vi "REFERECNE Dashboard Main.vi"() -> ()   [LabVIEW 2023]
uses:
  Shared Code/TypeDefs/ENUM RB_Drive Mode IND.ctl
  Shared Code/TypeDefs/Cluster_CMD_Direction Data.ctl
  Shared Code/TypeDefs/Cluster_Module Velocity-Direction-Rotations.ctl
  Shared Code/TypeDefs/Level_Velocity plus-minus 1.ctl
  Shared Code/TypeDefs/Dial_Compase heading unit circle CCW positive.ctl
  Shared Code/TypeDefs/ENUM RB_Feeder State.ctl
  Support/Utility/FP_Size VI to Decoration Simple.vi/TypeDefs_Utility/Cluster_FP Set.ctl
  Support/Utility/FP_Size VI to Decoration Simple.vi/TypeDefs_Utility/ENUM RB_Pos_Quadrant Position.ctl
  <vilib>/event_ctls.llb/eventvkey.ctl
  <vilib>/Utility/miscctls.llb/LVForegroundBackgroundColorsTypeDef.ctl
  dc37a527-230c-42ca-8007-a2fc15904402.vi
  b20e14a2-edb0-4227-a406-03726573f279.vi
  <vilib>/Rock Robotics/Network Tables/NT Read Numeric Array.vi
  <vilib>/Rock Robotics/WPI/Dashboard/WPI_DashboardLogging Global.vi
panel:
  in  "Camera Settings Right":T1={"Frame Rate"=30, "Compression"=30, "Size"=1, "DB Camera Config"=FALSE} {"Frame Rate" scale=1.0..30.0; "Compression" scale=100.0..-1.0; "Size" items=["640x480", "320x240", "160x120"]}
  in  "Camera Name Right":string(combo)="No Camera Selection"
  out "Camera Perf":string
  in  "Camera Settings":T1={"Frame Rate"=30, "Compression"=30, "Size"=1, "DB Camera Config"=FALSE} {"Frame Rate" scale=1.0..30.0; "Compression" scale=100.0..-1.0; "Size" items=["640x480", "320x240", "160x120"]}
  in  "TCP":refnum<k5>
  out "Robot IP":string
  out "Image Message":string="Timeout in Camera Communications"
  in  "Dashboard Tab":T2(tab)=enum."Custom"
  in  "Select Auto":string(combo)="Select Autonomous ..."
  out "NT Connection":bool
  out "MotorChart R":cluster{"Numeric":dbl, "Numeric":dbl}(graph)
  out "MotorChart L":cluster{"Numeric":dbl, "Numeric":dbl}(graph)
  out "MotorSliders R":cluster{"MotorSlide1":dbl, "MotorSlide2":dbl} {"MotorSlide2" scale=-1.0..1.0 scale format="%#_2e"; "MotorSlide1" scale=-1.0..1.0 scale format="%#_2e"}
  out "MotorSliders L":cluster{"MotorSlide1":dbl, "MotorSlide2":dbl} {"MotorSlide2" scale=-1.0..1.0 scale format="%#_2e"; "MotorSlide1" scale=-1.0..1.0 scale format="%#_2e"}
  out "JS1 Z":dbl(slide) scale=-1.0..1.0 scale format="%#_2e"
  out "JS1 Graph":cluster{"X":dbl, "Y":dbl}[](graph)
  out "JS1 Buttons":T3
  out "JS2 Z":dbl(slide) scale=-1.0..1.0 scale format="%#_2e"
  out "JS2 Graph":cluster{"X":dbl, "Y":dbl}[](graph)
  out "JS2 Buttons":T3
  out "Mode":T4(ring)=enum."Auto Disabled"
  out "Right Camera Perf":cluster{"Bandwidth (Mbps)":dbl, "FPS":dbl}
  out "Camera Image Right":T5(plugin-control)
  in  "DB/String 9":string
  in  "DB/String 8":string
  in  "DB/String 7":string
  in  "DB/String 6":string
  in  "DB/String 5":string
  in  "DB/String 4":string
  in  "DB/String 3":string
  in  "DB/String 2":string
  in  "DB/String 1":string
  in  "DB/String 0":string
  in  "DB/Slider 0":dbl(slide) scale=0.0..5.0
  in  "DB/Slider 1":dbl(slide) scale=0.0..5.0
  in  "DB/Slider 2":dbl(slide) scale=0.0..5.0
  in  "DB/Slider 3":dbl(slide) scale=0.0..5.0
  out "DB/LED 3":bool
  out "DB/LED 2":bool
  out "DB/LED 1":bool
  out "DB/LED 0":bool
  in  "DB/Button 3":bool
  in  "DB/Button 2":bool
  in  "DB/Button 1":bool
  in  "DB/Button 0":bool caption="New Name"
  in  "Max Speed (FPS)":dbl(slide)=2.0 min=0.0 max=10.0 step=0.1 scale=0.0..10.0
  out "Tube":string
  out "Drive State":bool=TRUE
  out "Feeder State":T6
  out "Shooter Speed":cluster{dbl, dbl, dbl}(slide) scale=0.0..4500.0 scale format="%#.0f"
  out "Compass":T7 scale format="%.3f"
  out "Comand Data":T8 {"Rotate(Yaw) CCW 1 CW -1" scale=1.0..-1.0; "Traverse"."Angle" scale format="%.3f"; "Traverse"."Velocity" scale=-1.0..1.0 scale format="%.1f"}
  out "Robot MODE":T11
  in  "CheckList":i32(listbox)
  out "Tree":string(tree)
  out "Camera Image":T5(plugin-control)
  out "Background":bool
  in  "Camera Name":string(combo)="No Camera Selection"
  # "HW"
  # "HW"
  # "Joysticks"
  # "Drive Motors"
  # "Front"
  # "Right"
  # "Left"
  # "Back"
  # "Setting"
  # "Right"
  # "Left"
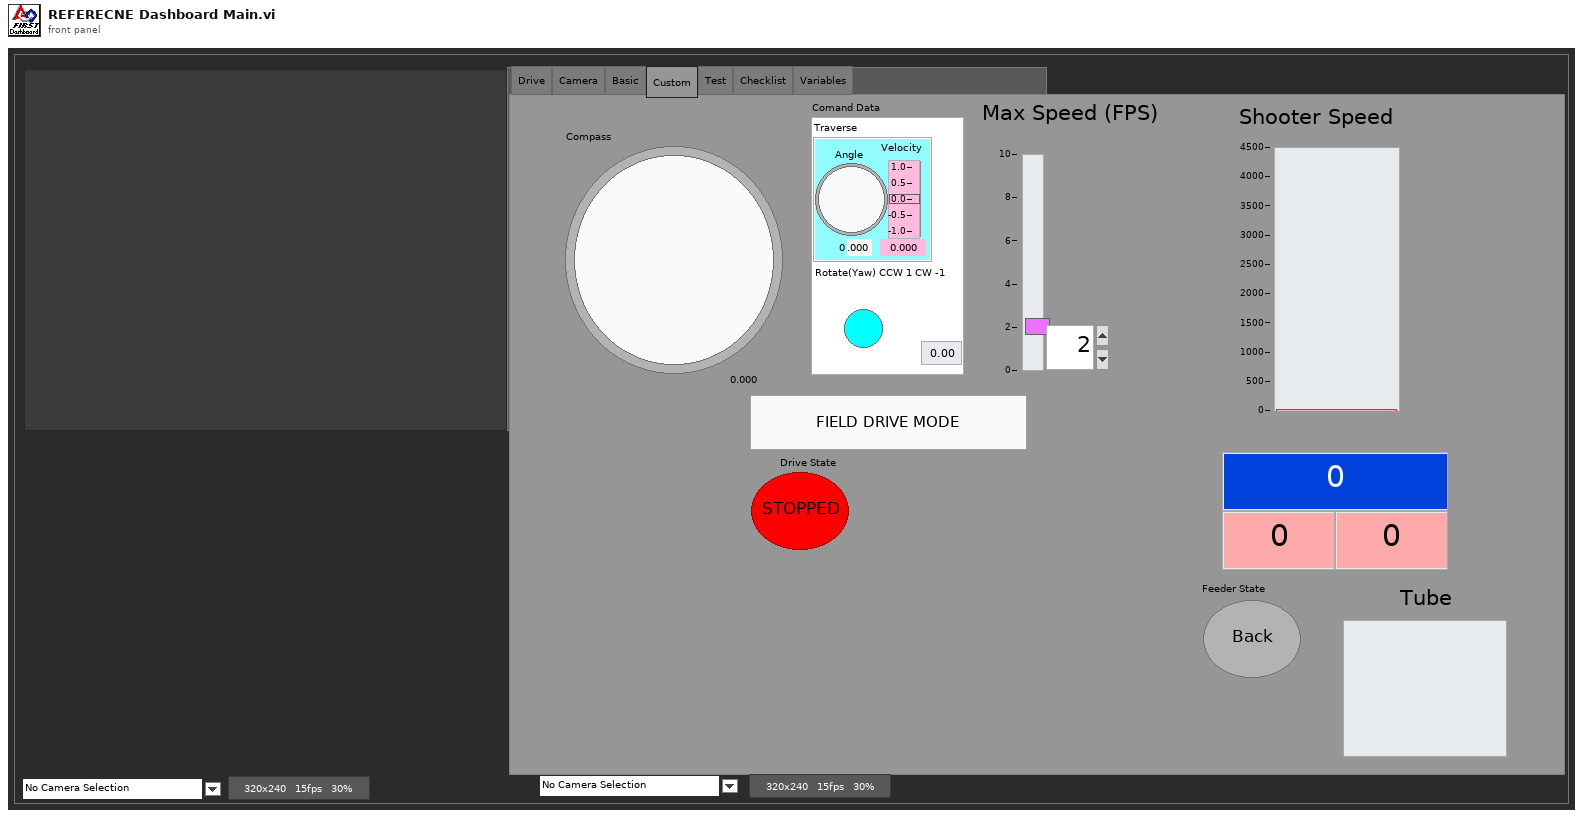
[diagram p1: front panel]
types:
  T1 = cluster{"Frame Rate":i32, "Compression":i32, "Size":u16, "DB Camera Config":bool}
  T2 = enum32{"Drive", "Camera", "Basic", "Custom", "Test", "Checklist", "Variables"}
  T3 = cluster{bool, bool, bool, bool, bool, bool, bool, bool, bool, bool, bool, bool}
  T4 = enum8{"Tele-Op Disabled", "Tele-Op Enabled", "Auto Disabled", "Auto Enabled", "Test Disabled", "Test Enabled", "Disconnected", "No Code", "E-Stop"}
  T5 = typedef "IMAQ Image.ctl" = refnum<image>
  T6 = typedef "ENUM RB_Feeder State.ctl" = enum32{"Back", "Reversing", "Shooting"}
  T7 = typedef "Dial_Compase heading unit circle CCW positive.ctl" = dbl
  T8 = typedef "Cluster_CMD_Direction Data.ctl" = cluster{"Traverse":T9, "Rotate(Yaw) CCW 1 CW -1":dbl}
  T9 = typedef "Cluster_Module Velocity-Direction-Rotations.ctl" = cluster{"Velocity":T10, "Angle":T7, "Rotations Count":dbl}
  T10 = typedef "Level_Velocity plus-minus 1.ctl" = dbl
  T11 = typedef "ENUM RB_Drive Mode IND.ctl" = enum32{"Field Drive Mode", "Robot Drive Mode", "Turrent Drive Mode"}
  T12 = typedef "Cluster_FP Set.ctl" = cluster{"Menu Bar":bool, "Position":T13, "Decoration index":i32, "border(px)":i32, "Monitor #":i32}
  T13 = typedef "ENUM RB_Pos_Quadrant Position.ctl" = enum32{"LFT-TOP", "MID-TOP", "RGT-TOP", "LFT-CTR", "MID-CTR", "RGT-CTR", "LFT-BOT", "MID-BOT", "RGT-BOT"}
  T14 = cluster{"Save Path":path, "Interval (s)":dbl, "Keep":i32}
  T15 = enum32{"Drive", "Camera", "Basic", "Custom", "Test", "Commands", "Checklist", "Variables"}
  T16 = typedef "Image Type" = u32
  T17 = typedef "LVForegroundBackgroundColorsTypeDef.ctl" = cluster{"Foreground Color":u32, "Background Color":u32}
  T18 = cluster{"Error Strings":string, "Disable Counts":cluster{u16, u16}, "Rail Faults":cluster{u16, u16, u16}, "Robot IP":string, "DB Mode":u8, "Event Info":cluster{"Name":string, "Type":u8, "Number":u16, "Replay":u8}}
  T19 = cluster{"Storage":cluster{"Disk Free":u64, "RAM Block":u32, "RAM free":u32}, "CPU Utilization":cluster{"CPU % ISR":sgl, "CPU % Time Crit":sgl, "CPU % Timed Str":sgl, "CPU % High":sgl, "CPU % Above":sgl, "CPU % Normal":sgl, "CPU % Low":sgl}, "CAN":cluster{"% Bus Utilization":sgl, "Bus Off Cnt":u32, "TX_FIFO Full Cnt":u32, "Receive Error Cnt":u8, "Transmit Error Cnt":u8}, "HID":cluster{"HID Outputs":u32, "Rumble Low":u16, "Rumble High":u16}[]}
  T20 = cluster{"Status bits":cluster{"Test Mode":bool, "Autonomous":bool, "Enabled":bool, "Code Start":bool, "Brownout":bool, "Reserved 2":bool, "Reserved 3":bool, "E-Stop":bool}, "Code Trace":cluster{"Disabled":bool, "TeleOp":bool, "Auto":bool, "Test":bool}, "Controller Type":enum16{"unknown", "cRIO", "roboRio"}, "Code?":enum16{"unknown", "noCode", "code"}, "Battery V":dbl}
  T21 = cluster{"Control Bits":cluster{"TestMode":bool, "Autonomous":bool, "Enabled":bool, "FMS Present":bool, bool, bool, bool, "E-Stop":bool}, "Team Station ":u8, "Countdown":sgl, "Joystick Values":cluster{"Axes":dbl[], "Buttons":bool[], "POVs":i16[]}[]}
  T22 = typedef "Cluster_Shooter Speed Data.ctl" = cluster{"Set":dbl, "Left":dbl, "Right":dbl}
  T23 = typedef "ENUM_Tube Wheel Positions.ctl" = enum16{"Unknown-None", "Tube Red A", "Tube Black B", "Tube Red C", "Tube Black D", "Tube Red E", "Tube Black F", "Load A-B", "Load B-C", "Load C-D", "Load D-E", "Load E-F", "Load F-A"}
  T24 = cluster{"Axes":dbl[], "Buttons":bool[], "POVs":i16[]}[]
  T25 = cluster{"Axes":dbl[], "Buttons":bool[], "POVs":i16[]}
  T26 = cluster{"Buttons[0]":bool, "Buttons[1]":bool, "Buttons[2]":bool, "Buttons[3]":bool, "Buttons[4]":bool, "Buttons[5]":bool, "Buttons[6]":bool, "Buttons[7]":bool, "Buttons[8]":bool, "Buttons[9]":bool, "Buttons[10]":bool, "Buttons[11]":bool}
  T27 = cluster{"Global Rectangle":i32[], "Contours":cluster{"Contour Type":u32, "ROI Type":u32, "Points":i32[]}[]}
  T28 = cluster{"Camera Name Right":string, string, "Saved DB Images Info":cluster{"Save Path":path, "Interval (s)":dbl, "Keep":i32}}
  T29 = cluster{"Camera Name":string, string, "Saved DB Images Info":cluster{"Save Path":path, "Interval (s)":dbl, "Keep":i32}}
  T30 = cluster{"Operation":enum16{"Update", "Clear"}, "Color Box":u32}[]
  T31 = typedef "eventvkey.ctl" = enum16{"ASCII", "Enter", "Return", "Shift", "Ctrl", "Alt", "Cmd", "Opt", "Caps", "NumLock", "Clear", "Break", "Up", "Down", "Left", "Right", "Insert", "Delete", "Home", "End", "PageUp", "PageDown", "Escape", "Help", "Pause", "ScrollLock", "F1", "F2", "F3", "F4", "F5", "F6", "F7", "F8", "F9", "F10", "F11", "F12", "F13", "F14", "F15", "F16", "F17", "F18", "F19", "F20", "F21", "F22", "F23", "F24", "Play", "VolumeUp", "VolumeDown", "Mute", "Two Byte Char"}
  T32 = cluster{"Shift":bool, "Ctrl":bool, "Alt":bool, "Cmd":bool, "Opt":bool}
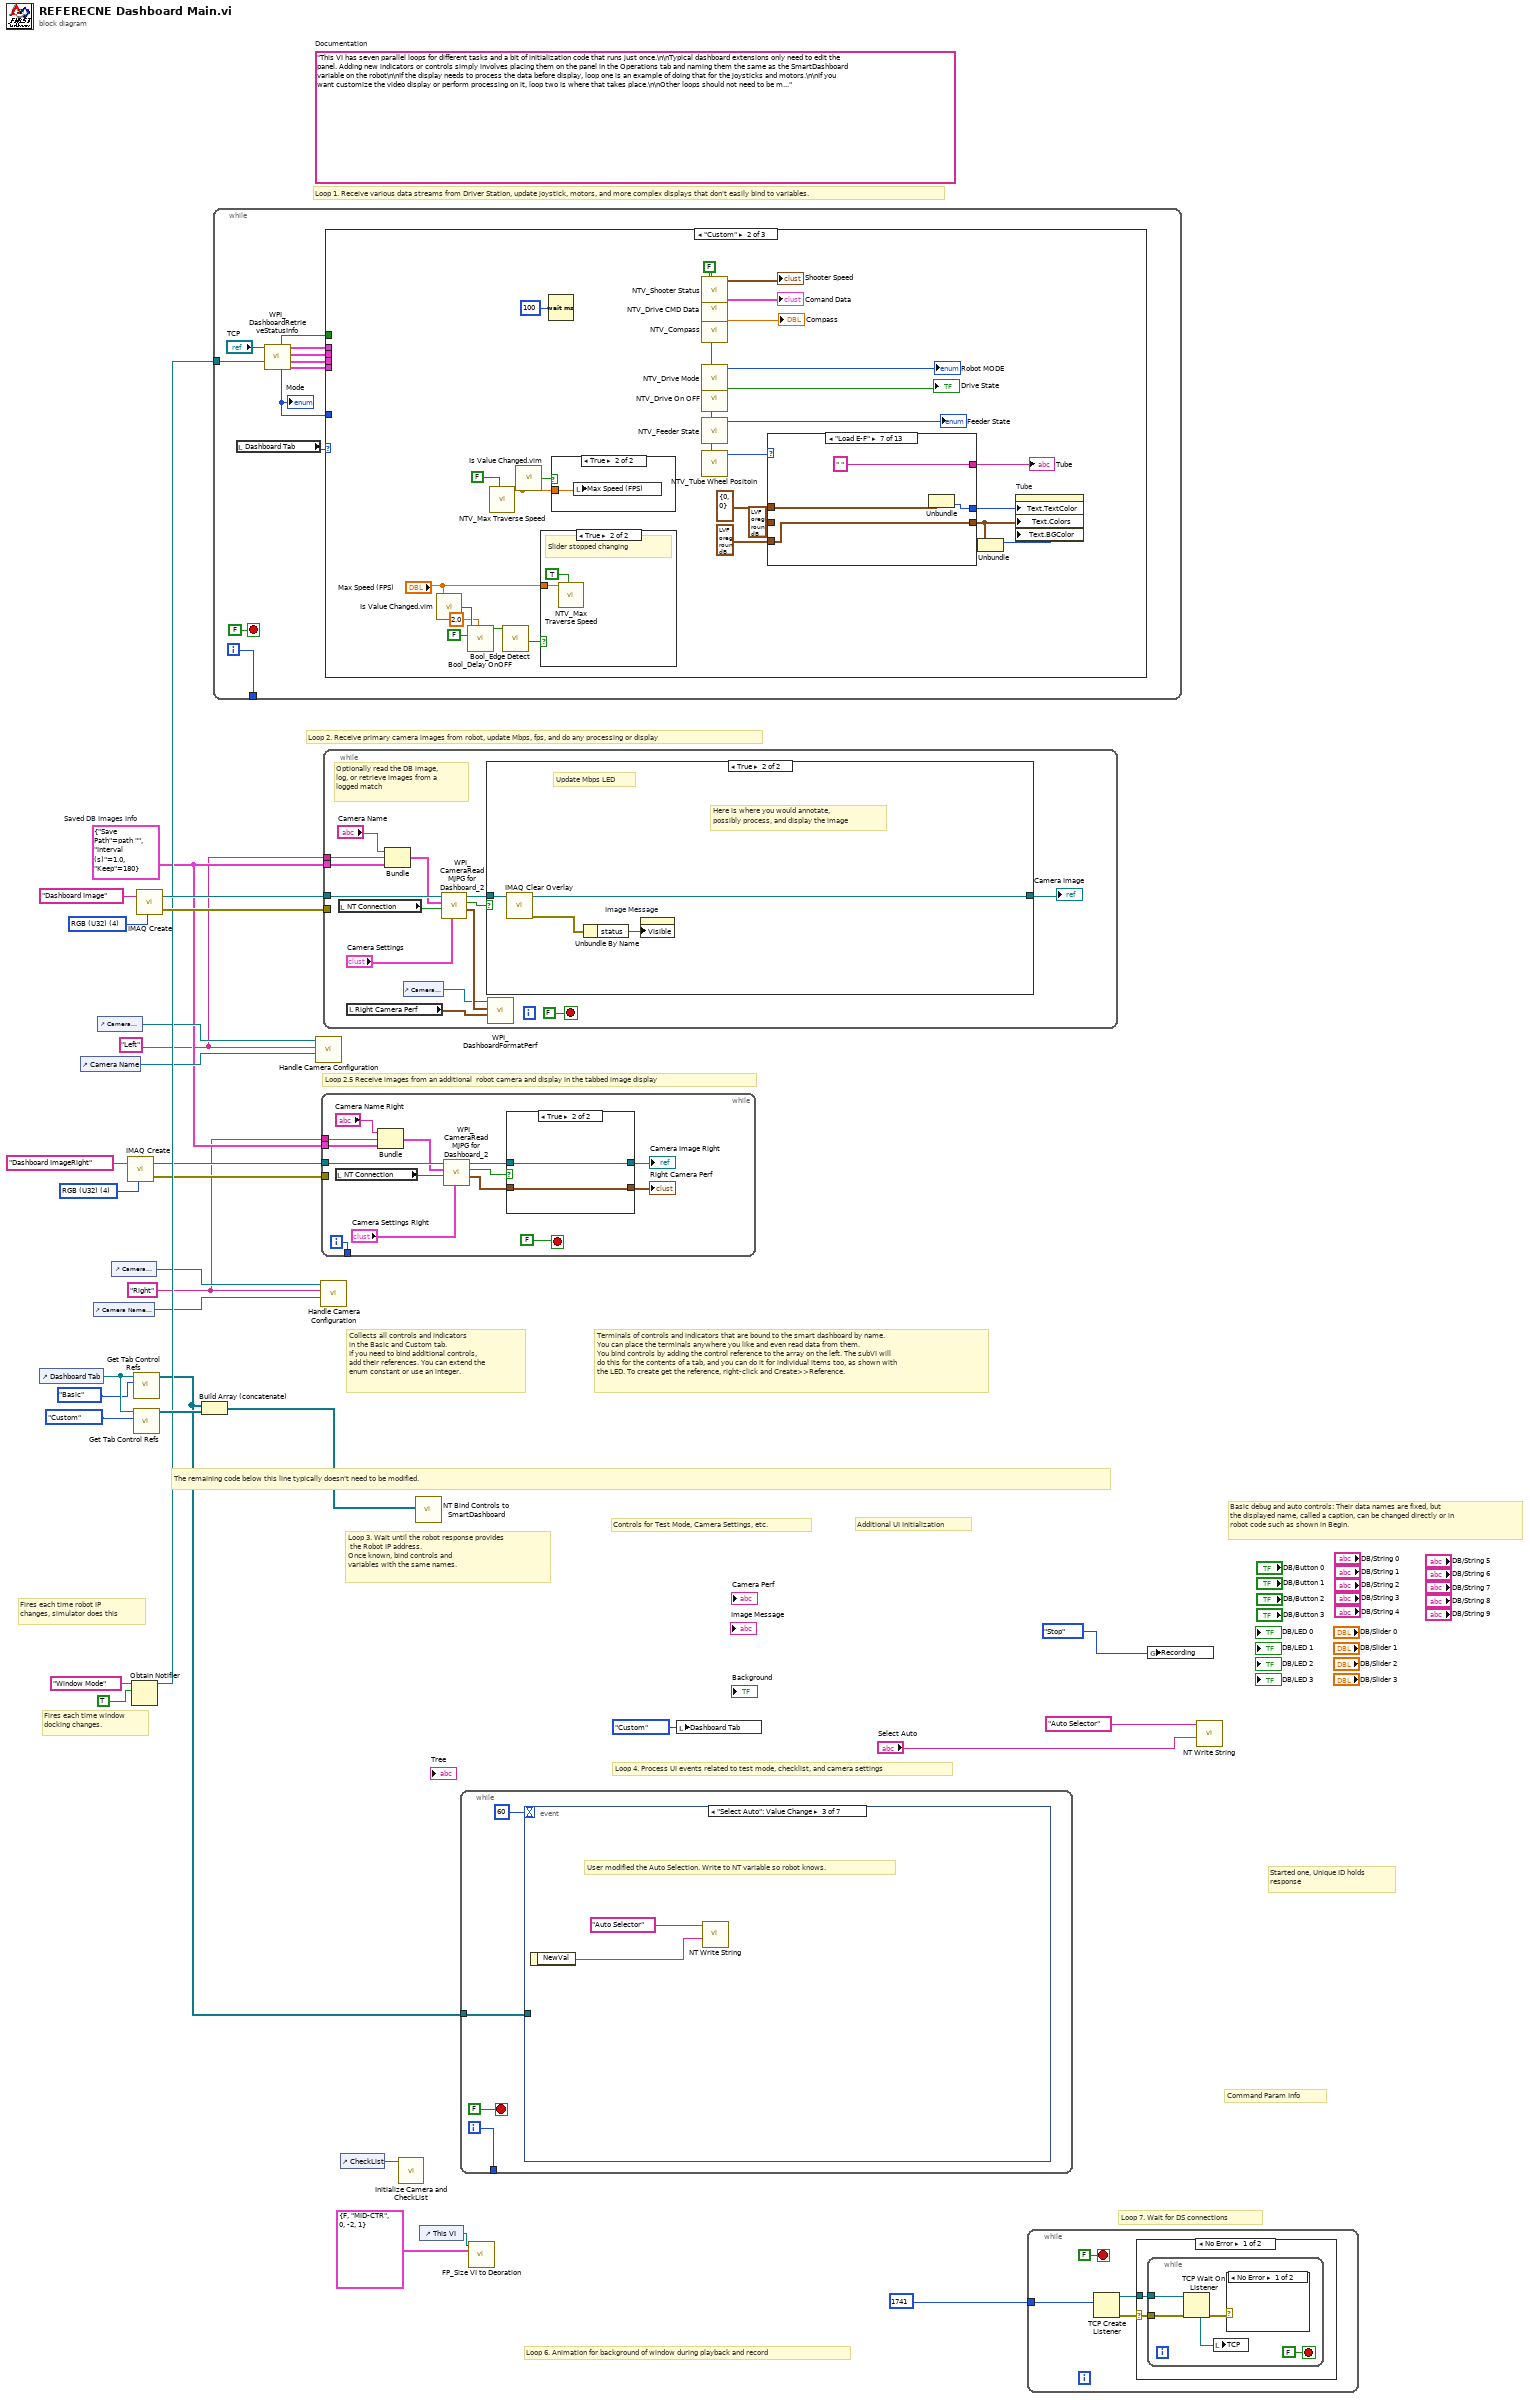
[diagram p0: block diagram]
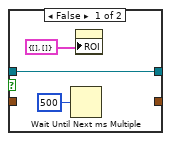
[diagram p2: hidden frame]
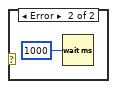
[diagram p3: hidden frame]
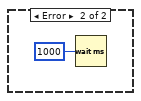
[diagram p4: hidden frame]
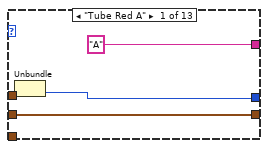
[diagram p8: hidden frame]
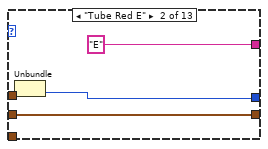
[diagram p9: hidden frame]
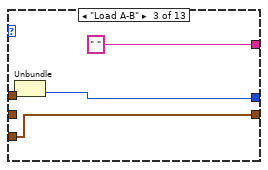
[diagram p10: hidden frame]
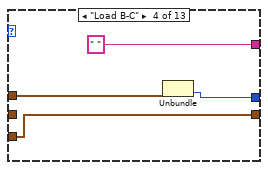
[diagram p11: hidden frame]
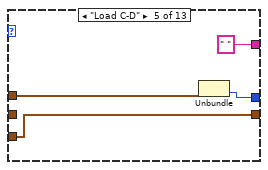
[diagram p12: hidden frame]
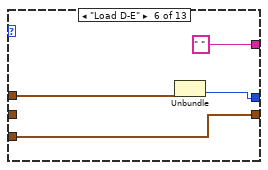
[diagram p13: hidden frame]
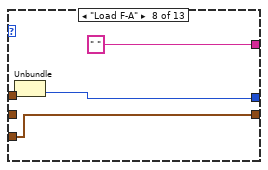
[diagram p14: hidden frame]
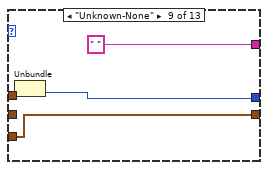
[diagram p15: hidden frame]
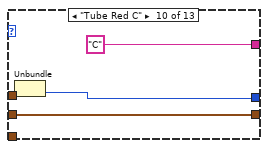
[diagram p16: hidden frame]
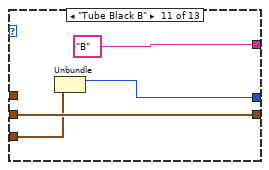
[diagram p17: hidden frame]
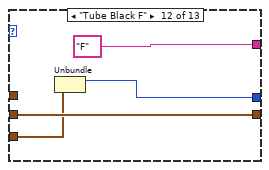
[diagram p18: hidden frame]
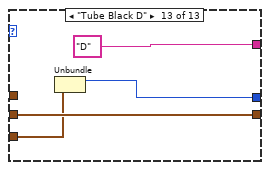
[diagram p19: hidden frame]
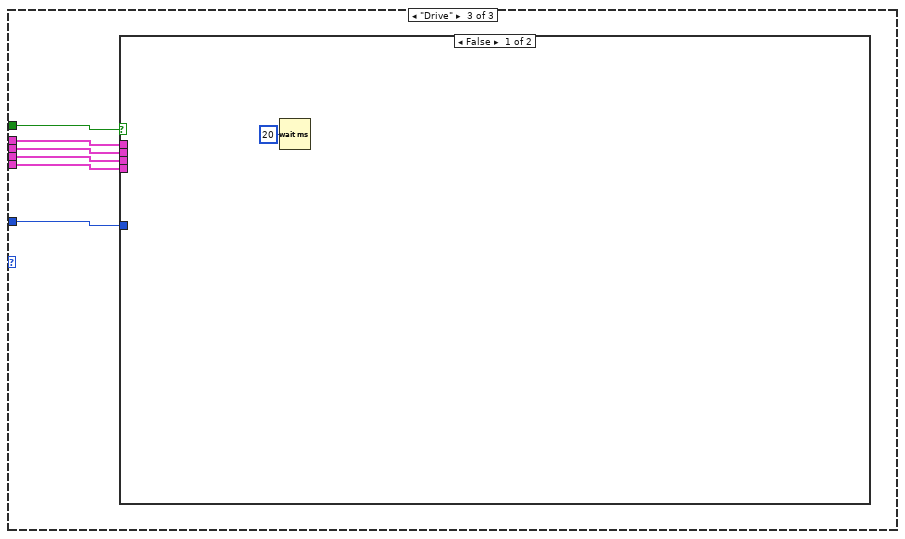
[diagram p20: hidden frame]
diagram:
  w7 = T14 {"Save Path"=path "", "Interval (s)"=1.0, "Keep"=180}  # Saved DB Images Info
  w6 = "Right"
  w5 = "Left"
  w14 = T16 4 items=["Grayscale (U8)", "Grayscale (I16)", "Grayscale (SGL)", "Complex (CSG)", "RGB (U32)", "HSL (U32)", "RGB (U64)"] ("Image Type")
  (unwired) "This VI has seven parallel loops for different tasks and a bit of initialization code that runs just once.\n\nTypical dashboard extensions only need to edit the panel. Adding new indicators or controls simply involves placing them on the panel in the Operations tab and naming them the same as the SmartDashboard variable on the robot\n\nIf the display needs to process the data before display, loop one is an example of doing that for the joysticks and motors.\n\nIf you want customize the video display or perform processing on it, loop two is where that takes place.\n\nOther loops should not need to be modified. They are pretty standard, and document the task they perform."  # Documentation
  w32 = T16 4 items=["Grayscale (U8)", "Grayscale (I16)", "Grayscale (SGL)", "Complex (CSG)", "RGB (U32)", "HSL (U32)", "RGB (U64)"] ("Image Type")
  # "Loop 2.5 Receive images from an additional  robot camera and display in the tabbed image display"
  # "Command Param Info"
  # "Started one, Unique ID holds\nresponse"
  # "Loop 7. Wait for DS connections"
  # "Basic debug and auto controls: Their data names are fixed, but\nthe displayed name, called a caption, can be changed directly or in\nrobot code such as shown in Begin."
  # "Controls for Test Mode, Camera Settings, etc."
  # "Additional UI Initialization"
  # "Loop 6. Animation for background of window during playback and record"
  # "Fires each time robot IP\nchanges, simulator does this"
  # "Fires each time window\ndocking changes."
  # "Collects all controls and indicators\nin the Basic and Custom tab.\nIf you need to bind additional controls,\nadd their references. You can extend the\nenum constant or use an integer."
  # "The remaining code below this line typically doesn't need to be modified."
  # "Loop 4. Process UI events related to test mode, checklist, and camera settings"
  # "Terminals of controls and indicators that are bound to the smart dashboard by name.\nYou can place the terminals anywhere you like and even read data from them.\nYou bind controls by adding the control reference to the array on the left. The subVI will\ndo this for the contents of a tab, and you can do it for individual items too, as shown with\nthe LED. To create get the reference, right-click and Create>>Reference."
  # "Loop 3. Wait until the robot response provides\n the Robot IP address.\nOnce known, bind controls and\nvariables with the same names."
  # "Loop 1. Receive various data streams from Driver Station, update joystick, motors, and more complex displays that don't easily bind to variables."
  # "Loop 2. Receive primary camera images from robot, update Mbps, fps, and do any processing or display"
  n1 = control-ref of="Dashboard Tab"() -> (w25:refnum<vi>)
  n2 = control-ref of="Camera Name"() -> (w19:refnum<vi>)
  n3 = control-ref of="Camera Name Right"() -> (w10:refnum<vi>)
  n4 = control-ref of="Camera Settings"() -> (w20:refnum<vi>)
  n5 = control-ref of="Camera Settings Right"() -> (w11:refnum<vi>)
  n6 = call "IMAQ Create"("Image Name"="Dashboard ImageRight", "Image Type"=w14) -> ("New Image"=w13:T5, "error out"=w12:errorcluster)  [unwired: 2 in, 1 out]
  n7 = Obtain Notifier(name (unnamed)="Window Mode", notification data type=TRUE) -> (notifier out=w22:refnum<notifier>)  [unwired: 2 in, 2 out]
  n8 = call <vilib>:"Get Tab Control Refs.vi"("Page Index"=T15."Basic" ("Dashboard Tab"), "TabControl in"=w25) -> ("ControlsOnPage"=w18:refnum<vi>[])  [unwired: 9 in]
  n9 = call <vilib>:"Get Tab Control Refs.vi"("Page Index"=T15."Custom" ("Dashboard Tab"), "TabControl in"=w25) -> ("ControlsOnPage"=w24:refnum<vi>[])  [unwired: 9 in]
  n10 = call "IMAQ Create"("Image Name"="Dashboard Image", "Image Type"=w32) -> ("New Image"=w30:T5, "error out"=w29:errorcluster)  [unwired: 2 in, 1 out]
  n11 = Build Array (concatenate)(w18, w24) -> (w4:refnum<vi>[])
  n12 = while {
    tunnel: [w42] -> _
    tunnel: w22 -> [w41]
    i -> [w42]
    stop <- FALSE stop-if-true
    n13 = local read "Dashboard Tab"() -> (w33:T2)
    n14 = call <vilib>:"WPI_DashboardRetrieveStatusInfo.vi"("Window Mode Notifier"=w41, "TCP Cnx"="TCP") -> ("Power and Errors"=w36:T18, "Robot Metrics"=w39:T19, "Status Info"=w40:T20, "Control Info"=w37:T21, "Robot Mode"=w35:T4, "Process?"=w38:bool)  [unwired: 4 in]
    "Mode" <- w35
    n15 = case shown="\"Custom\"" w33 {
      tunnel: w40 -> [_ _ w129]
      tunnel: w39 -> [_ _ w128]
      tunnel: w38 -> [_ _ w127]
      tunnel: w37 -> [_ _ w126]
      tunnel: w36 -> [_ _ w125]
      tunnel: w35 -> [_ _ w124]
      frame Default {
      }
      frame "Custom" {
        w46 = FALSE ("Read(f) Write(t)")
        n16 = call "Is Value Changed.vim"("value"="Max Speed (FPS)") -> ("changed or first call?"=w52:bool)
        n17 = call "Bool_Delay OnOFF.vi"("Delay Time(S)"=2.0, "Delay On(t) Off(f)"=FALSE, "Input"=w52) -> ("Output"=w49:bool)  [unwired: 7 in, 1 out]
        n18 = call "NTV_Max Traverse Speed.vi"("Read(f) Write(t)"=FALSE) -> ("MAx Traverse Speed FPS Out"=w44:dbl)  [unwired: 10 in]
        n19 = call "Bool_Edge Detect.vi"("Input/Set"=w49) -> ("Fall"=w48:bool)  [unwired: 7 in, 3 out]
        n20 = call "Is Value Changed.vim"("value"=w44) -> ("changed or first call?"=w45:bool)
        n21 = case shown="True" w48 {
          tunnel: "Max Speed (FPS)" -> [_ w70]
          frame False {
            # "no change or stil changing"
          }
          frame True {
            # "Slider stopped changing"
            n22 = call "NTV_Max Traverse Speed.vi"("Read(f) Write(t)"=TRUE, "MAx Tavers Speed FPS"=w70) -> ()  [unwired: 9 in, 1 out]
          }
        }
        n23 = Wait (ms)(milliseconds to wait=u32 100) -> ()  [unwired: 1 out]
        n24 = case shown="True" w45 {
          tunnel: w44 -> [_ w69]
          frame False {
          }
          frame True {
            n25 = local write "Max Speed (FPS)"(w69) -> ()
          }
        }
        n26 = call "NTV_Shooter Status.vi"("Read(f) Write(t)"=w46) -> ("Shooter Speed"=→"Shooter Speed":T22)  [unwired: 10 in]
        n27 = call "NTV_Drive CMD Data.vi"("Read(f) Write(t)"=w46) -> ("Comand Data Out"=→"Comand Data":T8)  [unwired: 10 in]
        n28 = call "NTV_Compass.vi"("Read(f) Write(t)"=w46) -> ("Compass Out"=→"Compass":T7)  [unwired: 10 in]
        n29 = call "NTV_Drive Mode.vi"("Read(f) Write(t)"=w46) -> ("Drive Mode"=→"Robot MODE":T11)  [unwired: 10 in]
        n30 = call "NTV_Drive On OFF.vi"("Read(f) Write(t)"=w46) -> ("Run Stop Out"=→"Drive State":bool)  [unwired: 10 in]
        n31 = call "NTV_Feeder State.vi"("Read(f) Write(t)"=w46) -> ("Feeder State Out"=→"Feeder State":T6)  [unwired: 10 in]
        n32 = call "NTV_Tube Wheel Positoin.vi"("Read(f) Write(t)"=w46) -> ("Feeder State Out"=w61:T23)  [unwired: 10 in]
        n33 = case shown="\"Load E-F\"" w61 {
          tunnel: T17 {"Foreground Color"=16711680, "Background Color"=16711680} ("Text.Colors") -> [w75 w79 _ _ _ _ _ _ _ w111 _ _ _]
          tunnel: T17 {"Foreground Color"=0, "Background Color"=0} ("Text.Colors") -> [w73 w77 w82 w86 w90 w94 w98 w102 w106 w109 w115 w119 w123]
          tunnel: [w75 w79 w80 w84 w88 w92 w96 w100 w104 w111 w115 w119 w123] -> w55
          tunnel: [w72 w76 w81 w85 w89 w93 w97 w101 w105 w108 w112 w116 w120] -> w58
          tunnel: ["A" ("Tube") "E" ("Tube") " " ("Tube") " " ("Tube") " " ("Tube") " " ("Tube") " " ("Tube") " " ("Tube") " " ("Tube") "C" ("Tube") "B" ("Tube") "F" ("Tube") "D" ("Tube")] -> w57
          tunnel: T17 {"Foreground Color"=16448250, "Background Color"=16448250} ("Text.Colors") -> [_ _ w80 w84 w88 w92 w96 w100 w104 _ w113 w117 w121]
          frame "Tube Red A" {
            n34 = Unbundle(w73) -> ("Background Color"=w72:u32)  [unwired: 1 out]
          }
          frame "Tube Red E" {
            n35 = Unbundle(w77) -> ("Background Color"=w76:u32)  [unwired: 1 out]
          }
          frame "Load A-B" {
            n36 = Unbundle(w82) -> ("Background Color"=w81:u32)  [unwired: 1 out]
          }
          frame "Load B-C" {
            n37 = Unbundle(w86) -> ("Background Color"=w85:u32)  [unwired: 1 out]
          }
          frame "Load C-D" {
            n38 = Unbundle(w90) -> ("Background Color"=w89:u32)  [unwired: 1 out]
          }
          frame "Load D-E" {
            n39 = Unbundle(w94) -> ("Background Color"=w93:u32)  [unwired: 1 out]
          }
          frame "Load E-F" {
            n40 = Unbundle(w98) -> ("Background Color"=w97:u32)  [unwired: 1 out]
          }
          frame "Load F-A" {
            n41 = Unbundle(w102) -> ("Background Color"=w101:u32)  [unwired: 1 out]
          }
          frame "Unknown-None" {
            n42 = Unbundle(w106) -> ("Background Color"=w105:u32)  [unwired: 1 out]
          }
          frame "Tube Red C" {
            n43 = Unbundle(w109) -> ("Background Color"=w108:u32)  [unwired: 1 out]
          }
          frame "Tube Black B" {
            n44 = Unbundle(w113) -> ("Foreground Color"=w112:u32)  [unwired: 1 out]
          }
          frame "Tube Black F" {
            n45 = Unbundle(w117) -> ("Foreground Color"=w116:u32)  [unwired: 1 out]
          }
          frame "Tube Black D" {
            n46 = Unbundle(w121) -> ("Foreground Color"=w120:u32)  [unwired: 1 out]
          }
        }
        "Tube" <- w57
        n47 = Unbundle(w55) -> ("Foreground Color"=w54:u32)  [unwired: 1 out]
        n48 = property on="Tube" class="Str"("Text.TextColor"=w58, "Text.Colors"=w55, "Text.BGColor"=w54) -> ()  [unwired: 2 in, 2 out]
      }
      frame "Drive" {
        n49 = case shown="False" w127 {
          tunnel: w129 -> [_ w154]
          tunnel: w128 -> [_ w153]
          tunnel: w126 -> [_ w152]
          tunnel: w125 -> [_ w151]
          tunnel: w124 -> [_ _]
          frame False {
            n50 = Wait (ms)(milliseconds to wait=u32 20) -> ()  [unwired: 1 out]
          }
          frame True {
            # "swap motors to match\ncharts and include battery"
            n51 = Unbundle By Name(w152) -> ("Joystick Values"=w142:T24)  [unwired: 1 out]
            n52 = Unbundle By Name(w153) -> ()  [unwired: 1 out]
            n53 = Unbundle By Name(w151) -> ("Robot IP"=→"Robot IP":string)
            n54 = Unbundle By Name(w154) -> ()  [unwired: 2 out]
            n55 = call-poly <vilib>:"NT Read Value.vi"("name"="RobotDrive Motors" ("Name")) -> ("value"=w132:dbl[])  [unwired: 8 in, 2 out]
            n56 = Index Array(array=w132, index #1=1, index #4=0) -> (element #1=w146:dbl, element #2=w147:dbl, element #3=w145:dbl, element #4=w150:dbl)  [unwired: 2 in]
            n57 = Index Array(array=w142) -> (element #1=w141:T25, element #2=w137:T25)  [unwired: 2 in]
            n58 = call "Prepare Joystick Data for Displays.vi"("Joystick Values"=w137) -> ("Buttons"=→"JS2 Buttons":T26, "Z Axis"=→"JS2 Z":dbl, "Cartesian Data"=→"JS2 Graph":cluster{"X axis":dbl, "X axis":dbl}[])  [unwired: 8 in]
            n59 = call "Prepare Joystick Data for Displays.vi"("Joystick Values"=w141) -> ("Buttons"=→"JS1 Buttons":T26, "Z Axis"=→"JS1 Z":dbl, "Cartesian Data"=→"JS1 Graph":cluster{"X axis":dbl, "X axis":dbl}[])  [unwired: 8 in]
            n60 = Bundle("Numeric"=w145, "Numeric"=w146) -> (→"MotorChart R" →"MotorSliders R":cluster{"Numeric":dbl, "Numeric":dbl})  [unwired: 1 in]
            n61 = Bundle("Numeric"=w147, "Numeric"=w150) -> (→"MotorChart L" →"MotorSliders L":cluster{"Numeric":dbl, "Numeric":dbl})  [unwired: 1 in]
          }
        }
      }
    }
  }
  n62 = call "Handle Camera Configuration.vi"("CameraNameRef"=w19, "Display Name"=w5, "ClusterRef"=w20) -> ()  [unwired: 9 in]
  n63 = call "Handle Camera Configuration.vi"("CameraNameRef"=w10, "Display Name"=w6, "ClusterRef"=w11) -> ()  [unwired: 9 in]
  n64 = while {
    tunnel: w13 -> [w168]
    tunnel: w12 -> [_]
    tunnel: [w164] -> _
    tunnel: w7 -> [w160]
    tunnel: w6 -> [w157]
    i -> [w164]
    stop <- FALSE stop-if-true
    n65 = local read "NT Connection"() -> (w161:bool)
    n66 = Bundle("Camera Name Right"="Camera Name Right", w157, "Saved DB Images Info"=w160) -> (w159:T28)  [unwired: 1 in]
    n67 = call <vilib>:"WPI_CameraRead MJPG for Dashboard_2.vi"("Camera Settings"="Camera Settings Right", "NT Connection"=w161, "Capture Info"=w159, "Image in"=w168) -> ("perf info"=w155:cluster{"Bandwidth (Mbps)":dbl, "fps":dbl}, "Active"=w163:bool, "Image\\ out"=w166:T5)  [unwired: 5 in]
    n68 = case shown="True" w163 {
      tunnel: w166 -> [w170 w173]
      tunnel: [w170 w173] -> w162
      tunnel: [_ w172] -> w156
      tunnel: w155 -> [_ w172]
      frame False {
        n69 = Wait Until Next ms Multiple(millisecond multiple=u32 500) -> ()  [unwired: 1 out]
        n70 = property on="Camera Image Right" class="ImageControl"("ROI"=T27 {"Global Rectangle"=[], "Contours"=[]}) -> ()  [unwired: 2 in, 2 out]
      }
      frame True {
      }
    }
    "Camera Image Right" <- w162
    "Right Camera Perf" <- w156
  }
  n71 = while {
    tunnel: w30 -> [w186]
    tunnel: w29 -> [_]
    tunnel: w7 -> [w180]
    tunnel: w5 -> [w177]
    stop <- FALSE stop-if-true
    # "Optionally read the DB image,\nlog, or retrieve images from a\nlogged match"
    n72 = local read "NT Connection"() -> (w181:bool)
    n73 = local read "Right Camera Perf"() -> (w175:cluster{"Bandwidth (Mbps)":dbl, "FPS":dbl})
    n74 = Bundle("Camera Name"="Camera Name", w177, "Saved DB Images Info"=w180) -> (w179:T29)  [unwired: 1 in]
    n75 = control-ref of="Camera Perf"() -> (w174:refnum<vi>)
    n76 = call <vilib>:"WPI_CameraRead MJPG for Dashboard_2.vi"("Camera Settings"="Camera Settings", "NT Connection"=w181, "Capture Info"=w179, "Image in"=w186) -> ("perf info"=w176:cluster{"Bandwidth (Mbps)":dbl, "fps":dbl}, "Active"=w184:bool, "Image\\ out"=w185:T5)  [unwired: 5 in]
    n77 = case shown="True" w184 {
      tunnel: w185 -> [w189 w192]
      tunnel: [w189 w191] -> w182
      frame False {
        # "Sleep for 500ms"
        n78 = property on="Camera Image" class="ImageControl"("ROI"=T27 {"Global Rectangle"=[], "Contours"=[]}) -> ()  [unwired: 2 in, 2 out]
        n79 = Wait Until Next ms Multiple(millisecond multiple=u32 500) -> ()  [unwired: 1 out]
      }
      frame True {
        # "Here is where you would annotate,\npossibly process, and display the image"
        # "Update Mbps LED"
        n80 = call "IMAQ Clear Overlay"("Image"=w192) -> ("error out"=w193:errorcluster, "Image Out"=w191:T5)  [unwired: 2 in, 7 out]
        n81 = Unbundle By Name(w193) -> ("status"=w194:bool)
        n82 = property on="Image Message" class="Str"("Visible"=w194) -> ()  [unwired: 2 in, 2 out]
      }
    }
    "Camera Image" <- w182
    n83 = call <vilib>:"WPI_DashboardFormatPerf.vi"("Right Camera Perf"=w175, "Performance"=w176, "String in"=w174) -> ()  [unwired: 9 in]
  }
  n84 = control-ref of="CheckList"() -> (w23:refnum<vi>)
  n85 = call "Initialize Camera and CheckList.vi"("ListBox in"=w23) -> ()  [unwired: 11 in]
  n86 = call <vilib>:"NT Bind Controls to SmartDashboard.vi"("Bound Control Refs"=w4) -> ()  [unwired: 11 in]
  n87 = control-ref of="This VI"() -> (w1:refnum<vi>)
  n88 = while {
    tunnel: [w196] -> _
    tunnel: w18 -> [w195]
    i -> [w196]
    stop <- FALSE stop-if-true
    n89 = event shown="[2] \"Select Auto\": Value Change" {
      selector: _ -> [_ _ _ _ _ _ _]
      dyn-events: _ -> [_ _ _ _ _ _ _]
      timeout: u32 60 ("milliseconds to wait") -> [_ _ _ _ _ _ _]
      tunnel: w195 -> [w199 _ _ _ _ _ _]
      event Timeout {
        n90 = event-data() -> ()  [unwired: 1 in, 1 out]
        n91 = local read "Mode"() -> (w202:T4)
        n92 = case shown="\"Test\"" "Dashboard Tab" {
          tunnel: "TestMode/Automatic/" ("Name Pattern") -> [_ _ _ _]
          tunnel: T30 [{"Operation"=enum."Clear", "Color Box"=14013909}, {"Operation"=enum."Clear", "Color Box"=14013909}, {"Operation"=enum."Clear", "Color Box"=14013909}, {"Operation"=enum."Clear", "Color Box"=14013909}, {"Operation"=enum."Update", "Color Box"=14013909}, {"Operation"=enum."Update", "Color Box"=16777215}, {"Operation"=enum."Clear", "Color Box"=14013909}, {"Operation"=enum."Clear", "Color Box"=14013909}, {"Operation"=enum."Clear", "Color Box"=14013909}] -> [_ _ _ _]
          tunnel: w202 -> [_ _ _ _]
          tunnel: u32[] [15790320, 15790320, 15790320, 15790320, 16777215, 16777215, 15790320, 15790320, 15790320] -> [_ _ _ _]
          tunnel: w199 -> [_ w206 _ _]
          frame "Custom", Default {
          }
          frame "Basic" {
            n93 = call <vilib>:"WPI_DashboardUpdateNames.vi"("Controls on Tab"=w206) -> ()  [unwired: 11 in]
          }
          frame "Test" {
          }
          frame "Variables" {
            w209 = string[] ["CameraPublisher", "Usage", "DB"]  # Items to initially close
            n94 = First Call?() -> (First Call?: T/F=w210:bool)
            n95 = control-ref of="Tree"() -> (w211:refnum<vi>)
            n96 = Select(t=w209, s=w210, f=string[] []) -> (s? t:f=w207:string[])
            n97 = call <vilib>:"NT Read and Format Entries as Tree.vi"("Tags to  Close"=w207, "Tree Refnum"=w211) -> ()  [unwired: 8 in, 2 out]
          }
        }
        n98 = call <vilib>:"Connextion Info.vi"() -> ("Connected"=→"NT Connection":bool)  [unwired: 10 in, 1 out]
      }
      event "Select Auto": Mouse Enter {
        # "Populate the combo box with the list of autonomous options"
        n99 = event-data() -> ()  [unwired: 1 in, 1 out]
        n100 = call <vilib>:"NT Read String Array.vi"("name"="Auto List" ("Name")) -> ("value"=w212:string[])  [unwired: 8 in, 2 out]
        n101 = property on="Select Auto" class="CmbBox"("Strings[]"=w212) -> ()  [unwired: 2 in, 2 out]
      }
      event "Select Auto": Value Change {
        # "User modified the Auto Selection. Write to NT variable so robot knows."
        n102 = event-data() -> ("NewVal"=w214:string)  [unwired: 1 in]
        n103 = call <vilib>:"NT Write String.vi"("value"=w214, "name"="Auto Selector" ("Name")) -> ()  [unwired: 9 in, 1 out]
      }
      event "CheckList": Double Click {
        # "Shift clears all"
        # "Update symbols on the listbox"
        n104 = event-data() -> ("PlatMods.Shift"=w216:bool, "Row"=w218:i32)  [unwired: 1 in]
        n105 = case shown="True" w216 {
          tunnel: w218 -> [w222 _]
          tunnel: 1 -> [w221 _]
          frame False {
            n106 = property on="CheckList" class="LstBox (strict)"() -> ("Item Symbols"=w220:i32[])  [unwired: 2 in, 2 out]
            n107 = Replace Array Subset(array=w220, new element=w221, index=w222) -> (w219:i32[])
            n108 = property on="CheckList" class="LstBox (strict)"("Item Symbols"=w219) -> ()  [unwired: 2 in, 2 out]
          }
          frame True {
            w223 = 0 ("Top Row")
            n109 = property on="CheckList" class="LstBox (strict)"() -> ("Number of Rows"=w225:u32)  [unwired: 2 in, 2 out]
            n110 = Initialize Array(0, w225) -> (w224:i32[])
            n111 = property on="CheckList" class="LstBox (strict)"("Top Row"=w223, "Value"=w223, "Item Symbols"=w224) -> ()  [unwired: 2 in, 2 out]
          }
        }
      }
      event "CheckList": Key Down {
        # "Update symbols on the listbox\nLeft and right keys check and uncheck"
        n112 = event-data() -> ("VKey"=w228:T31)  [unwired: 1 in]
        n113 = case shown="\"Left\", \"Right\"" w228 {
          selector: w228 -> [w233 _]
          tunnel: eventvkey."Left" ("VKey") -> [w231 _]
          frame "Left", "Right" {
            n114 = Equal?(x=w231, y=w233) -> (x = y?=w232:bool)
            n115 = Select(t=0, s=w232, f=1) -> (s? t:f=w234:i32)
            n116 = property on="CheckList" class="LstBox (strict)"() -> ("Item Symbols"=w237:i32[])  [unwired: 2 in, 2 out]
            n117 = Replace Array Subset(array=w237, new element=w234, index="CheckList") -> (w236:i32[])
            n118 = property on="CheckList" class="LstBox (strict)"("Item Symbols"=w236) -> ()  [unwired: 2 in, 2 out]
          }
          frame Default {
          }
        }
      }
      event Panel Close {
        # "Abort playback window and ourself"
        n119 = event-data() -> ()  [unwired: 1 in, 4 out]
        n120 = invoke class="VI" method="Abort VI"() -> ()  [unwired: 3 in, 3 out]
      }
      event "Tree": Double Click {
        n121 = event-data() -> ("PlatMods"=w243:T32, "Tag"=w240:string)  [unwired: 1 in]
        n122 = Unbundle(w243) -> ("Shift"=w242:bool)  [unwired: 4 out]
        n123 = String Subset(string=w240, length (rest)=1 ("length (rest)")) -> (substring=w239:string)  [unwired: 1 in]
        n124 = Not(x=w242) -> (.not. x?=w241:bool)
        n125 = case shown="\"/\"" w239 {
          tunnel: w240 -> [_ w245]
          tunnel: w241 -> [_ w244]
          frame Default {
          }
          frame "/" {
            n126 = call <vilib>:"NT Update Persistence.vi"("Persistence"=w244, "Name"=w245) -> ()  [unwired: 9 in, 1 out]
          }
        }
      }
    }
  }
  n127 = call "FP_Size VI to Deoration.vi"("FPSet"=T12 {"Menu Bar"=FALSE, "Position"=enum."MID-CTR", "Decoration index"=0, "border(px)"=-2, "Monitor #"=1}, "VI Ref"=w1) -> ()  [unwired: 8 in, 2 out]
  n128 = local write "Dashboard Tab"(T2."Custom" ("Dashboard Tab")) -> ()
  n129 = while {
    tunnel: u16 1741 ("timeout ms (25000)") -> [w247]
    stop <- FALSE stop-if-true
    n130 = TCP Create Listener(10:w247) -> (0:w246:errorcluster, 3:w248:refnum<k5>)  [unwired: 4 in, 1 out]
    n131 = case shown="No Error" w246 {
      selector: w246 -> [w250 _]
      tunnel: w248 -> [w251 _]
      frame No Error {
        n132 = while {
          tunnel: w251 -> [w254]
          tunnel: w250 -> [w253]
          stop <- FALSE stop-if-true
          n133 = TCP Wait On Listener(8:w253, 11:w254) -> (0:w255:errorcluster, 4:w256:refnum<k5>)  [unwired: 2 in, 3 out]
          n134 = local write "TCP"(w256) -> ()
          n135 = case shown="No Error" w255 {
            frame No Error {
            }
            frame Error {
              n136 = Wait (ms)(milliseconds to wait=u32 1000) -> ()  [unwired: 1 out]
            }
          }
        }
      }
      frame Error {
        n137 = Wait (ms)(milliseconds to wait=u32 1000) -> ()  [unwired: 1 out]
      }
    }
  }
  n138 = global write "WPI_DashboardLogging Global.vi" "Recording"(enum32{"Stop", "Record", "Playback"}."Stop" ("Rec Mode")) -> ()
  n139 = call <vilib>:"NT Write String.vi"("value"="Select Auto", "name"="Auto Selector" ("Name")) -> ()  [unwired: 9 in, 1 out]
